vi "Build Metadata Names.vi"(10 "Chassis Name":string) -> (0 "Modbus Wfm Hdr":string, 1 "Modbus Wfm":string, 2 "Wfm Hdr":string, 3 "Wfm":string, 4 "Down":string)   [LabVIEW 2012]
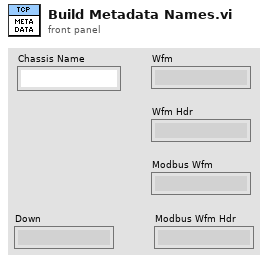
[diagram p1: front panel]
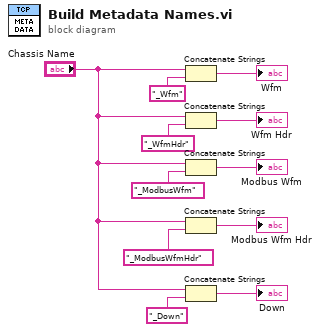
[diagram p0: block diagram]
diagram:
  n1 = Concatenate Strings("Chassis Name", "_Wfm") -> (→"Wfm":string)
  n2 = Concatenate Strings("Chassis Name", "_WfmHdr") -> (→"Wfm Hdr":string)
  n3 = Concatenate Strings("Chassis Name", "_ModbusWfm") -> (→"Modbus Wfm":string)
  n4 = Concatenate Strings("Chassis Name", "_ModbusWfmHdr") -> (→"Modbus Wfm Hdr":string)
  n5 = Concatenate Strings("Chassis Name", "_Down") -> (→"Down":string)
